vi "FTW-VAR-Attributes-DeleteRegexMatches.vi"(8 "error in":errorcluster, 9 "Force Literal Match?":bool, 10 "Regex Match for Attributes":string, 11 "Variant":variant) -> (0 "error out":errorcluster, 1 "Num Attributes Deleted":i16, 2 "Attributes Deleted":string[](array[string]), 3 "Variant out":variant)   [LabVIEW 2012]
panel:
  # "Inputs"
  # "Outputs"
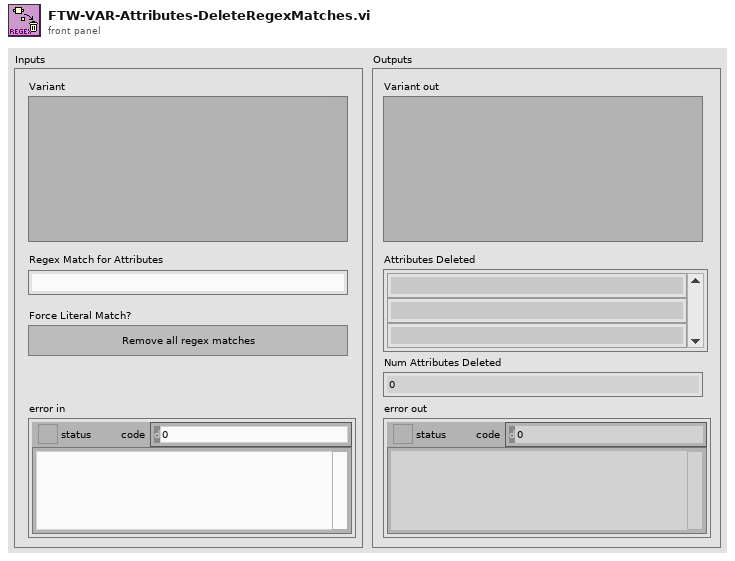
[diagram p1: front panel]
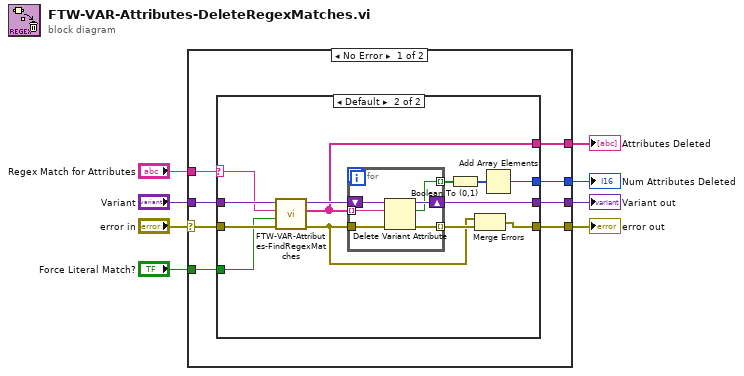
[diagram p0: block diagram]
diagram:
  n1 = case shown="No Error" "error in" {
    selector: "error in" -> [w11 w38]
    tunnel: "Variant" -> [w16 w39]
    tunnel: [w15 w39] -> w7
    tunnel: "Force Literal Match?" -> [w14 _]
    tunnel: [w13 w38] -> w5
    tunnel: "Regex Match for Attributes" -> [w12 _]
    tunnel: [w10 _] -> w1
    tunnel: [w9 _] -> w2
    frame No Error {
      n2 = case shown="Default" w12 {
        selector: w12 -> [_ w22]
        tunnel: w16 -> [w18 w25]
        tunnel: [w18 w31] -> w15
        tunnel: w14 -> [_ w21]
        tunnel: w11 -> [w17 w23]
        tunnel: [w17 w29] -> w13
        tunnel: [_ w26] -> w10
        tunnel: [_ w19] -> w9
        frame "" {
        }
        frame Default {
          n3 = call "FTW-VAR-Attributes-FindRegexMatches.vi"("error in"=w23, "Force Literal Match?"=w21, "Regex Match for Attributes"=w22, "Variant"=w25) -> ("error out"=w20:errorcluster, "Matching Attributes"=w19:string[], "Variant out"=w24:variant)  [unwired: 4 in, 1 out]
          n4 = for {
            tunnel: [w36] -> w30 mode=indexing
            shift-right: [w37] -> w31
            shift-left: w24 -> [w35]
            tunnel: w20 -> [w34]
            tunnel: w19 -> [w32] mode=indexing
            tunnel: [w33] -> w28 mode=indexing
            n5 = Delete Variant Attribute(4:w34, 6:w32, 7:w35) -> (0:w36:errorcluster, 2:w33:bool, 3:w37:variant)
          }
          n6 = Boolean To (0,1)(Boolean=w28) -> (0, 1=w27:i16[])
          n7 = Merge Errors(w20, w30) -> (w29:errorcluster)
          n8 = Add Array Elements(numeric array=w27) -> (sum=w26:i16)
        }
      }
    }
    frame Error {
    }
  }
  "error out" <- w5
  "Variant out" <- w7
  "Attributes Deleted" <- w2
  "Num Attributes Deleted" <- w1
